vi "Populate Actual Values.vi"(8 "error in":errorcluster, 11 "UI Actor in":refnum<class "UI Actor.lvclass">) -> (0 "error out":errorcluster, 3 "UI Actor out":refnum<class "UI Actor.lvclass">)   [LabVIEW 2019, in "UI Actor.lvlib" / "UI Actor.lvclass"]
uses:
  UI Actor.lvclass
  UI Actor.lvclass/UI Actor.ctl
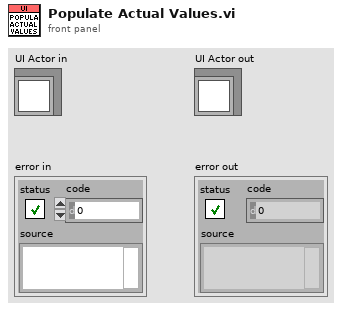
[diagram p1: front panel]
types:
  T1 = map{path, refnum<class "Electronic Datasheet.lvclass">}
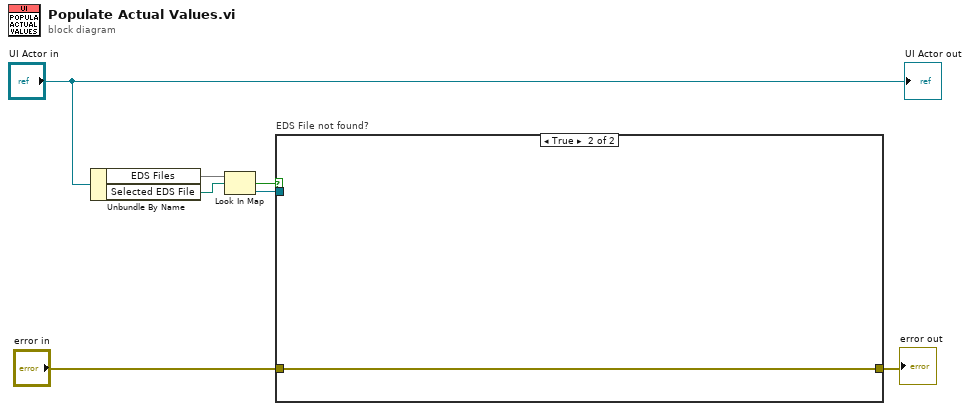
[diagram p0: block diagram]
diagram:
  n1 = Unbundle By Name("UI Actor in") -> ("EDS Files"=w7:T1, "Selected EDS File"=w6:path)
  n2 = Look In Map(map=w7, key=w6) -> (key not found?=w4:bool, value=w3:refnum<class "Electronic Datasheet.lvclass">)  [unwired: 1 in]
  n3 = case "EDS File not found?" shown="True" w4 {
    tunnel: w3 -> [_ _]
    tunnel: "error in" -> [w8 w9]
    tunnel: [w8 w9] -> w1
    frame False {
    }
    frame True {
    }
  }
  "error out" <- w1
  "UI Actor out" <- "UI Actor in"
